vi "solar_qtimer Set (Delay).vi"(8 "error in (no error)":errorcluster, 10 "Delay (-1)":i32=-1, 11 "QTimer Name":string) -> (0 "error out":errorcluster)   [LabVIEW 2018]
doc: "[DEPRECIATED] This sets the delay of the QTimer by name."
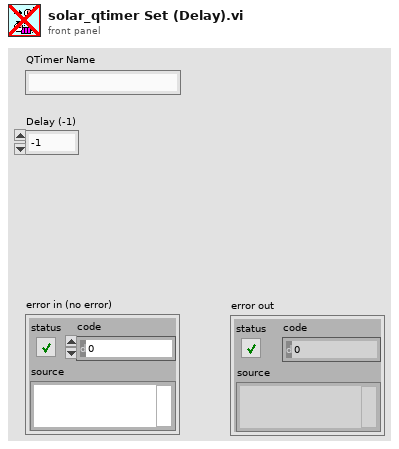
[diagram p1: front panel]
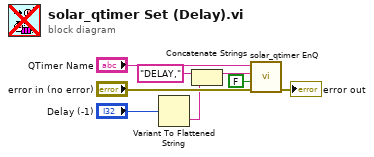
[diagram p0: block diagram]
diagram:
  n1 = Variant To Flattened String(Variant="Delay (-1)") -> (data string=w3:string)  [unwired: 1 out]
  n2 = Concatenate Strings("DELAY," ("CMD (\"\")"), w3) -> (w4:string)
  n3 = call "solar_qtimer EnQ.vi"("error in (no error)"="error in (no error)", "Create if not found? (F)"=FALSE, "CMD (\"\")"=w4, "QTimer Name"="QTimer Name") -> ("error out"=→"error out":errorcluster)  [unwired: 5 in, 2 out]
